vi "Compressor Latch.vi"(1 "Change?":bool) -> (0 "Value":bool)   [LabVIEW 2014]
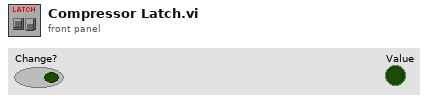
[diagram p1: front panel]
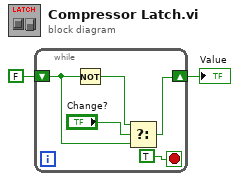
[diagram p0: block diagram]
diagram:
  n1 = while {
    shift-right: [w5] -> w1
    shift-left: FALSE -> [w4]
    stop <- TRUE stop-if-true
    n2 = Not(x=w4) -> (.not. x?=w3:bool)
    n3 = Select(t=w3, s="Change?", f=w4) -> (s? t:f=w5:bool)
  }
  "Value" <- w1
